vi "nanostage-check.vi"(4 "error in":errorcluster, 5 "axis set values":dbl[](array[numeric]), 7 "Axes to move":string[](array[string])) -> (0 "error out":errorcluster, 1 "parameters not ok":bool, 2 "moving":bool, 3 "get Values":cluster{"postion":dbl[], "status":bool[]})   [LabVIEW 2015]
panel:
  out "position error":dbl[](array[numeric])
  in  "threshold [nm]":i8=100 min=0 max=100 step=1 format="±%.0f"
  # "3D piezo nano stage"
  # "closed loop active?"
  # "check position [µm]"
  # "pos. accuracy [nm]"
  # "x-axis"
  # "y-axis"
  # "z-axis"
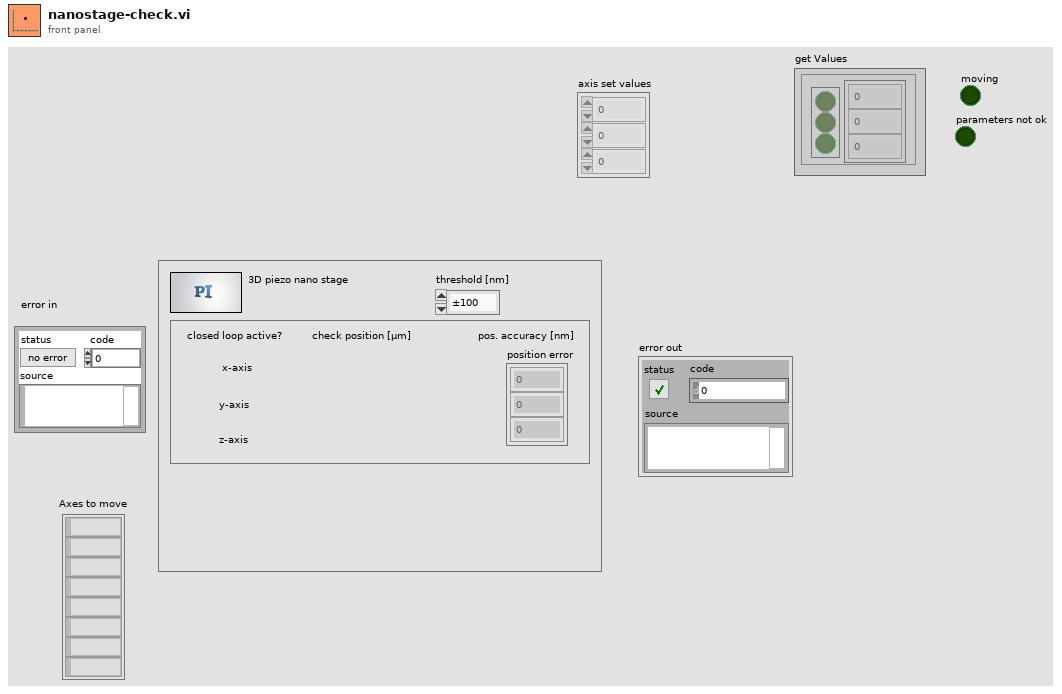
[diagram p1: front panel]
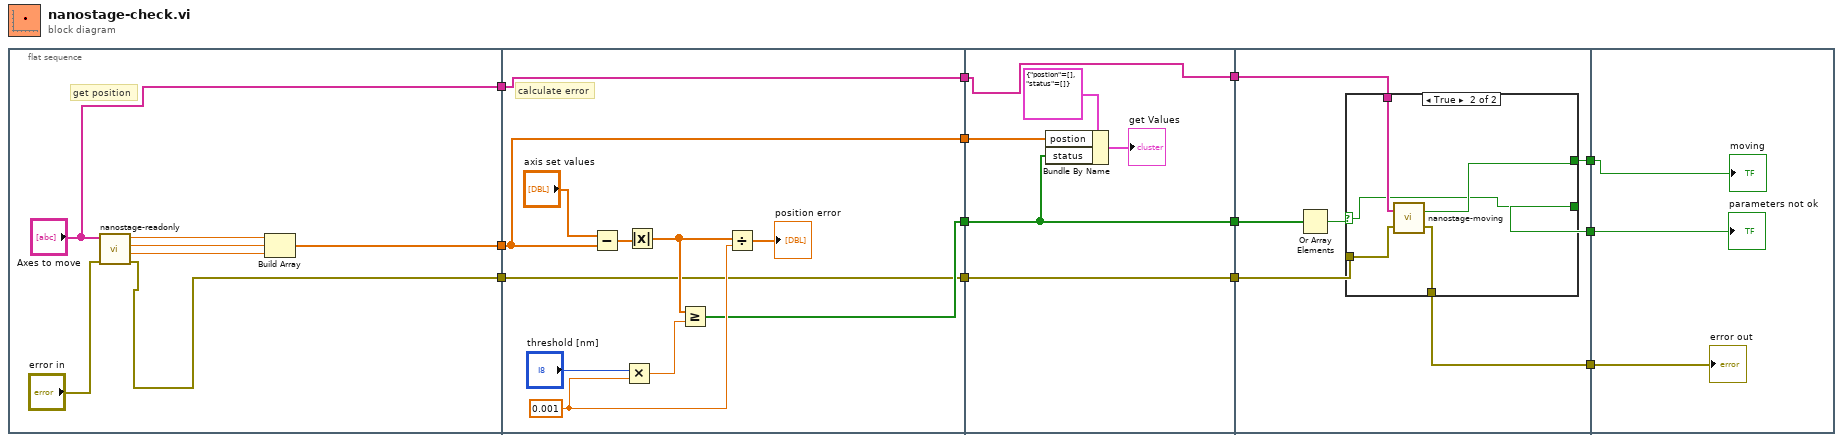
[diagram p0: block diagram]
diagram:
  n1 = flat-sequence {
    tunnel: [w17] -> w13
    tunnel: ["Axes to move"] -> w9
    tunnel: [w14] -> w6
    tunnel: w13 -> [w23]
    tunnel: [w24] -> w12
    tunnel: [w23] -> w10
    tunnel: w9 -> [w22]
    tunnel: [w22] -> w7
    tunnel: w6 -> [w21]
    tunnel: [w21] -> w5
    tunnel: w12 -> [w36]
    tunnel: [w36] -> w11
    tunnel: w10 -> [w37]
    tunnel: [w33] -> w8
    tunnel: w7 -> [w33]
    tunnel: w5 -> [w32]
    tunnel: [w32] -> w4
    tunnel: w11 -> [w44]
    tunnel: w8 -> [w42]
    tunnel: w4 -> [w41]
    tunnel: [w40] -> w3
    tunnel: [w39] -> w2
    tunnel: [w38] -> w1
    tunnel: w3 -> [w54]
    tunnel: w2 -> [w53]
    tunnel: w1 -> [w52]
    frame #0 {
      # "get position"
      n2 = call "nanostage-readonly.vi"("error in"="error in", "Axes to move"="Axes to move") -> ("error out"=w14:errorcluster, "position-z"=w18:dbl, "position-y"=w19:dbl, "position-x"=w20:dbl)  [unwired: 2 in]
      n3 = Build Array(w20, w19, w18) -> (w17:dbl[])
    }
    frame #1 {
      w25 = 0.001
      # "calculate error"
      n4 = Subtract(x="axis set values", y=w23) -> (x-y=w30:dbl[])
      n5 = Multiply(x="threshold [nm]", y=w25) -> (x*y=w26:dbl)
      n6 = Absolute Value(x=w30) -> (abs(x)=w28:dbl[])
      n7 = Greater Or Equal?(x=w28, y=w26) -> (x >= y?=w24:bool[])
      n8 = Divide(x=w28, y=w25) -> (x/y=→"position error":dbl[])
    }
    frame #2 {
      n9 = Bundle By Name(cluster=cluster{"postion":dbl[], "status":bool[]} {"postion"=[], "status"=[]} ("get Values"), "postion"=w37, "status"=w36) -> (→"get Values":cluster{"postion":dbl[], "status":bool[]})
    }
    frame #3 {
      n10 = Or Array Elements(Boolean array=w44) -> (logical OR=w43:bool)
      n11 = case shown="True" w43 {
        selector: w43 -> [w45 w47]
        tunnel: w42 -> [_ w51]
        tunnel: w41 -> [w46 w50]
        tunnel: [w46 w49] -> w40
        tunnel: [w45 w47] -> w39
        tunnel: [w45 w48] -> w38
        frame False {
        }
        frame True {
          n12 = call "nanostage-moving.vi"("error in"=w50, "Axes to query"=w51) -> ("error out"=w49:errorcluster, "moving"=w48:bool)
        }
      }
    }
    frame #4 {
      "parameters not ok" <- w53
      "error out" <- w54
      "moving" <- w52
    }
  }
